vi "Configure Instrument.vi"(0 "RFSG Session In":refnum<k15>, 5 "SG Configuration":T1={"SelectedPorts"="", "Reference Clock Source"="PXI_CLK", "Carrier Frequency (Hz)"=1000000000.0, "DUT Average Input Power (dBm)"=-10.0, "External Attenuation (dB)"=0.0, "LO Sharing Mode"=enum."Automatic"} {"Carrier Frequency (Hz)" format="%#_6p"}, 11 "error in (no error)":errorcluster) -> (4 "RFSG Session Out":refnum<k15>, 15 "error out":errorcluster)   [LabVIEW 2019, in "SG.lvlib"]
doc: "Configures common instrument settings for generation."
uses:
  SG.lvlib
  Typedefs/Instrument Configuration.ctl
  <instrlib>/niRFSG/niRFSG.llb/niRFSG Ref Clock Sources.ctl
  Common/Local Oscillator Sharing Mode.ctl
  Common/Common.lvlib
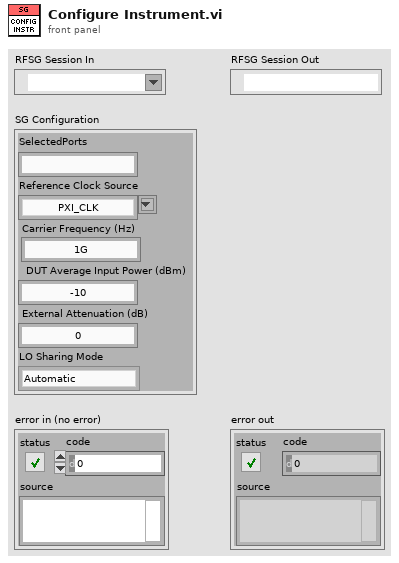
[diagram p1: front panel]
types:
  T1 = typedef "SG.lvlib/Instrument Configuration.ctl" = cluster{"SelectedPorts":string, "Reference Clock Source":T2, "Carrier Frequency (Hz)":dbl, "DUT Average Input Power (dBm)":dbl, "External Attenuation (dB)":dbl, "LO Sharing Mode":T3}
  T2 = typedef "niRFSG Ref Clock Sources.ctl" = string
  T3 = typedef "Common.lvlib/Local Oscillator Sharing Mode.ctl" = enum16{"Automatic", "None"}
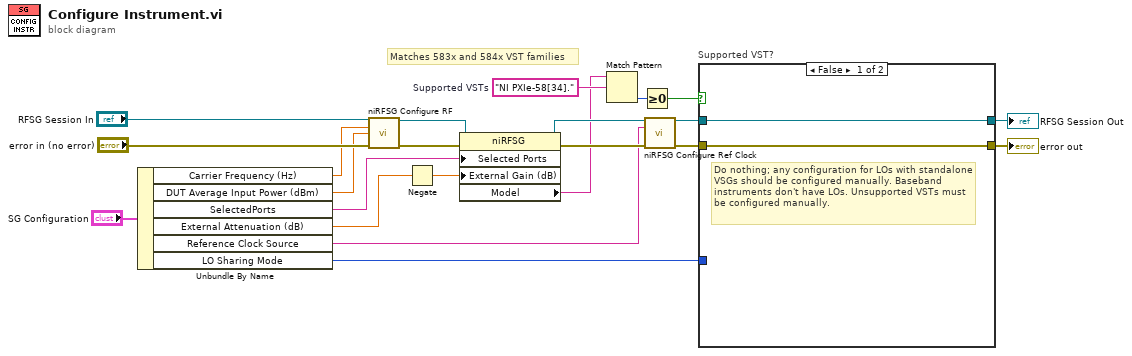
[diagram p0: block diagram]
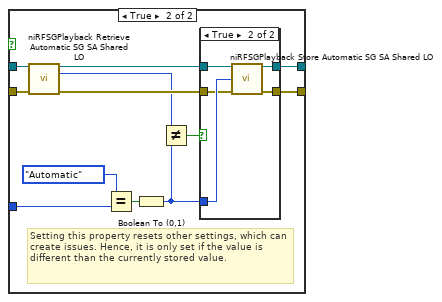
[diagram p2: hidden frame]
diagram:
  w7 = "NI PXIe-58[34]."  # Supported VSTs
  # "Matches 583x and 584x VST families"
  n1 = Unbundle By Name("SG Configuration") -> ("Carrier Frequency (Hz)"=w18:dbl, "DUT Average Input Power (dBm)"=w17:dbl, "SelectedPorts"=w11:string, "External Attenuation (dB)"=w14:dbl, "Reference Clock Source"=w13:T2, "LO Sharing Mode"=w1:T3)
  n2 = call <instrlib>:"niRFSG Configure RF.vi"("instrument handle"="RFSG Session In", "frequency (Hz)"=w18, "power level (dBm)"=w17, "error in"="error in (no error)") -> ("instrument handle out"=w16:refnum<k15>, "error out"=w21:errorcluster)  [unwired: 10 in]
  n3 = Negate(x=w14) -> (-x=w12:dbl)
  n4 = property class="niRFSG"(reference=w16, error in=w21, "Selected Ports"=w11, "External Gain (dB)"=w12) -> (reference out=w15:refnum<k15>, error out=w20:errorcluster, "Model"=w4:string)
  n5 = Match Pattern(string=w4, regular expression=w7) -> (offset past match=w6:i32)  [unwired: 1 in, 3 out]
  n6 = Greater Or Equal To 0?(x=w6) -> (x >= 0?=w5:bool)
  n7 = call <instrlib>:"niRFSG Configure Ref Clock.vi"("instrument handle"=w15, "ref clock source"=w13, "error in"=w20) -> ("instrument handle out"=w9:refnum<k15>, "error out"=w8:errorcluster)  [unwired: 11 in]
  n8 = case "Supported VST?" shown="False" w5 {
    tunnel: [w24 w33] -> w3
    tunnel: w8 -> [w23 w36]
    tunnel: [w23 w32] -> w2
    tunnel: w9 -> [w24 w29]
    tunnel: w1 -> [_ w35]
    frame False {
      # "Do nothing; any configuration for LOs with standalone VSGs should be configured manually. Baseband instruments don't have LOs. Unsupported VSTs must be configured manually."
    }
    frame True {
      # "Setting this property resets other settings, which can create issues. Hence, it is only set if the value is different than the currently stored value."
      n9 = call <instrlib>:"niRFSGPlayback Retrieve Automatic SG SA Shared LO.vi"("instrument handle in"=w29, "error in"=w36) -> ("instrument handle out"=w28:refnum<k15>, "automatic SG SA shared LO"=w27:i32, "error out"=w30:errorcluster)  [unwired: 11 in]
      n10 = Equal?(x=Local_Oscillator_Sharing_Mode."Automatic" ("LO Sharing Mode"), y=w35) -> (x = y?=w34:bool)
      n11 = Boolean To (0,1)(Boolean=w34) -> (0, 1=w26:i16)
      n12 = Not Equal?(x=w27, y=w26) -> (x != y?=w25:bool)
      n13 = case shown="True" w25 {
        tunnel: w26 -> [_ w43]
        tunnel: [w38 w42] -> w33
        tunnel: [w37 w41] -> w32
        tunnel: w30 -> [w37 w40]
        tunnel: w28 -> [w38 w39]
        frame False {
        }
        frame True {
          n14 = call <instrlib>:"niRFSGPlayback Store Automatic SG SA Shared LO.vi"("instrument handle in"=w39, "automatic SG SA shared LO"=w43, "error in"=w40) -> ("instrument handle out"=w42:refnum<k15>, "error out"=w41:errorcluster)  [unwired: 11 in]
        }
      }
    }
  }
  "error out" <- w2
  "RFSG Session Out" <- w3
